vi "To JSON.vi"(8 "error in":errorcluster, 11 "Theme Config in":refnum<class "Theme Config.lvclass">) -> (0 "error out":errorcluster, 2 "JSON":string, 3 "Theme Config out":refnum<class "Theme Config.lvclass">)   [LabVIEW 2021, in "Theme Config.lvclass"]
uses:
  Theme Config.lvclass
  Theme Config.lvclass/Theme Config.ctl
  51456f3c-de2e-4236-b56d-21e9e34e3997.vi
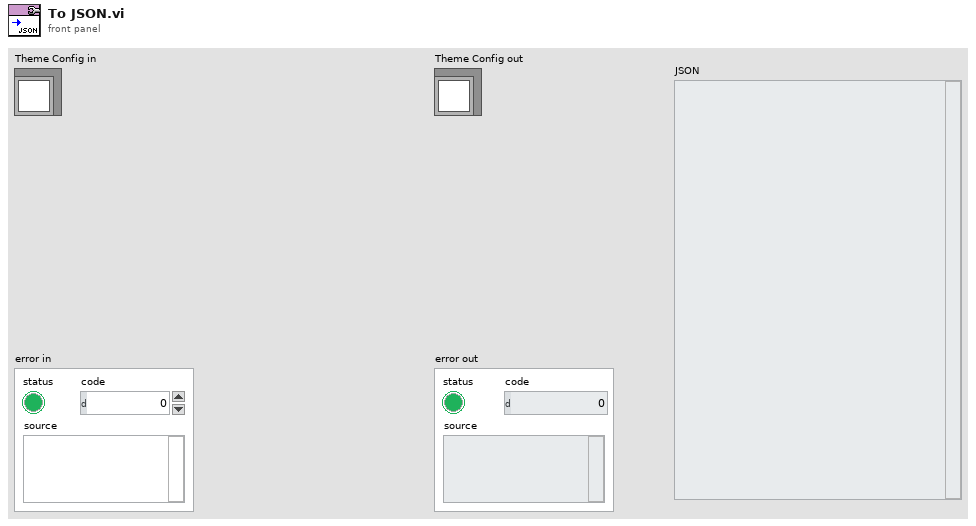
[diagram p1: front panel]
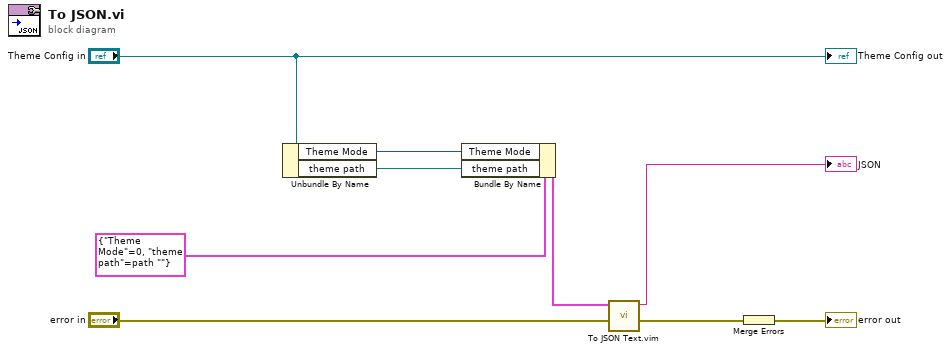
[diagram p0: block diagram]
diagram:
  n1 = Unbundle By Name("Theme Config in") -> ("Theme Mode"=w5:u16, "theme path"=w4:path)
  n2 = Bundle By Name(cluster=cluster{"Theme Mode":u16, "theme path":path} {"Theme Mode"=0, "theme path"=path ""} ("Cluster of class private data"), "Theme Mode"=w5, "theme path"=w4) -> (w2:cluster{"Theme Mode":u16, "theme path":path})
  n3 = call "To JSON Text.vim"("error in (no error)"="error in", "Anything"=w2) -> ("error out"=w3:errorcluster, "<JSON>"=→"JSON":string)  [unwired: 8 in]
  n4 = Merge Errors(w3) -> (→"error out":errorcluster)
  "Theme Config out" <- "Theme Config in"
